vi "get_phase_shift.vi"(8 "error in (no error)":errorcluster, 11 "TrajectoryTS090820Circular2D in":refnum<class "TrajectoryTS090820Circular2D.lvclass">) -> (0 "error out":errorcluster, 2 "Phase shift":dbl, 3 "TrajectoryTS090820Circular2D out":refnum<class "TrajectoryTS090820Circular2D.lvclass">)   [LabVIEW 2010, in "TrajectoryTS090820Circular2D.lvclass"]
uses:
  TrajectoryTS090820Circular2D.lvclass
  TrajectoryTS090820Circular2D.lvclass/TrajectoryTS090820Circular2D.ctl
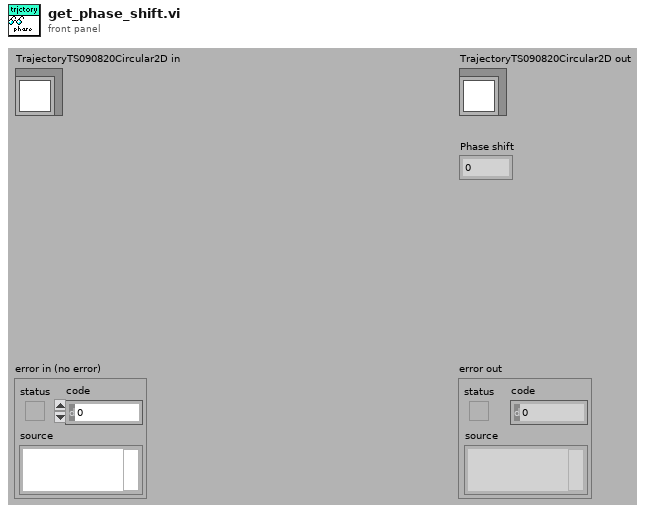
[diagram p1: front panel]
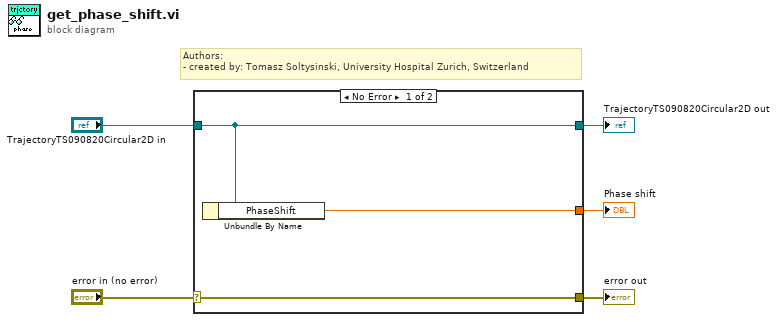
[diagram p0: block diagram]
diagram:
  # "Authors: \n- created by: Tomasz Soltysinski, University Hospital Zurich, Switzerland"
  n1 = case shown="No Error" "error in (no error)" {
    selector: "error in (no error)" -> [w8 w9]
    tunnel: [w8 w9] -> w4
    tunnel: [w7 w10] -> w2
    tunnel: "TrajectoryTS090820Circular2D in" -> [w7 w10]
    tunnel: [w6 _] -> w1
    frame No Error {
      n2 = Unbundle By Name(w7) -> ("PhaseShift"=w6:dbl)
    }
    frame Error {
    }
  }
  "error out" <- w4
  "TrajectoryTS090820Circular2D out" <- w2
  "Phase shift" <- w1
